vi "GetBoard.vi"(8 "error in (no error)":errorcluster, 11 "Game in":refnum<class "Game.lvclass">) -> (0 "error out":errorcluster, 2 "TronviewGame.lvlib:Board.lvclass":refnum<class "Board.lvclass">, 3 "Game out":refnum<class "Game.lvclass">)   [LabVIEW 2015, in "TronviewGame.lvlib" / "Game.lvclass"]
uses:
  Game.lvclass
  Board/Board.lvclass
  Game.lvclass/Game.ctl
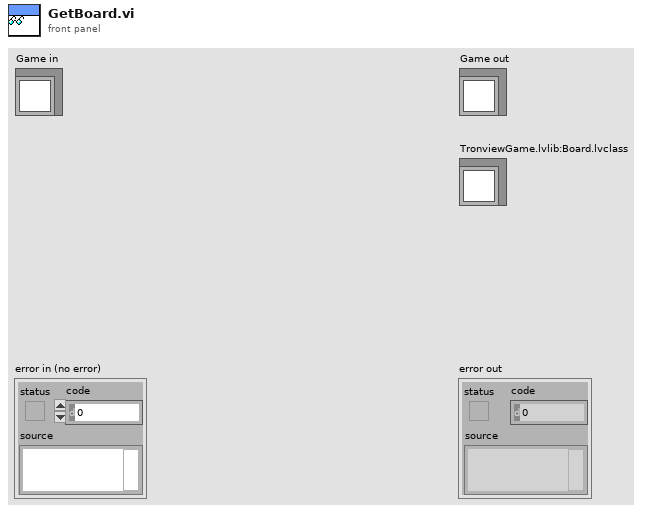
[diagram p1: front panel]
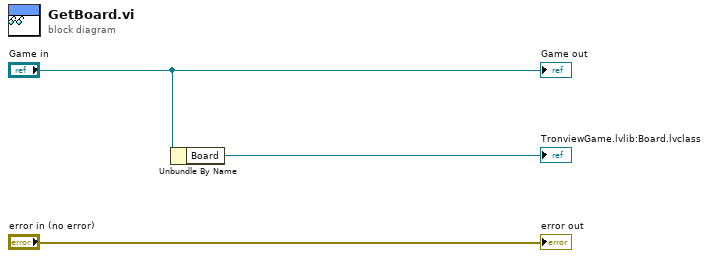
[diagram p0: block diagram]
diagram:
  n1 = Unbundle By Name("Game in") -> ("Board"=→"TronviewGame.lvlib:Board.lvclass":refnum<class "Board.lvclass">)
  "error out" <- "error in (no error)"
  "Game out" <- "Game in"
